vi "test-Vision-Utils-Test1.vi"() -> (3 "All Passed":bool)   [LabVIEW 2019]
uses:
  <vilib>/Rock Robotics/WPI/ThirdParty/JAS_Junk/TrajLib/Trajectory_Library.lvlib
panel:
  out "Dist To Targ 4":bool
  out "Dist To Targ 3":bool
  out "Dist To Targ 2":bool
  out "Dist To Targ 1":bool
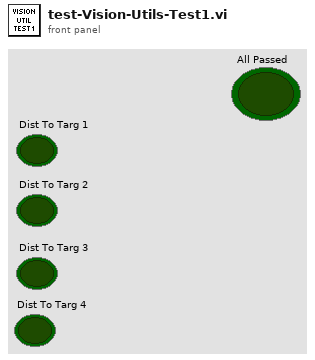
[diagram p1: front panel]
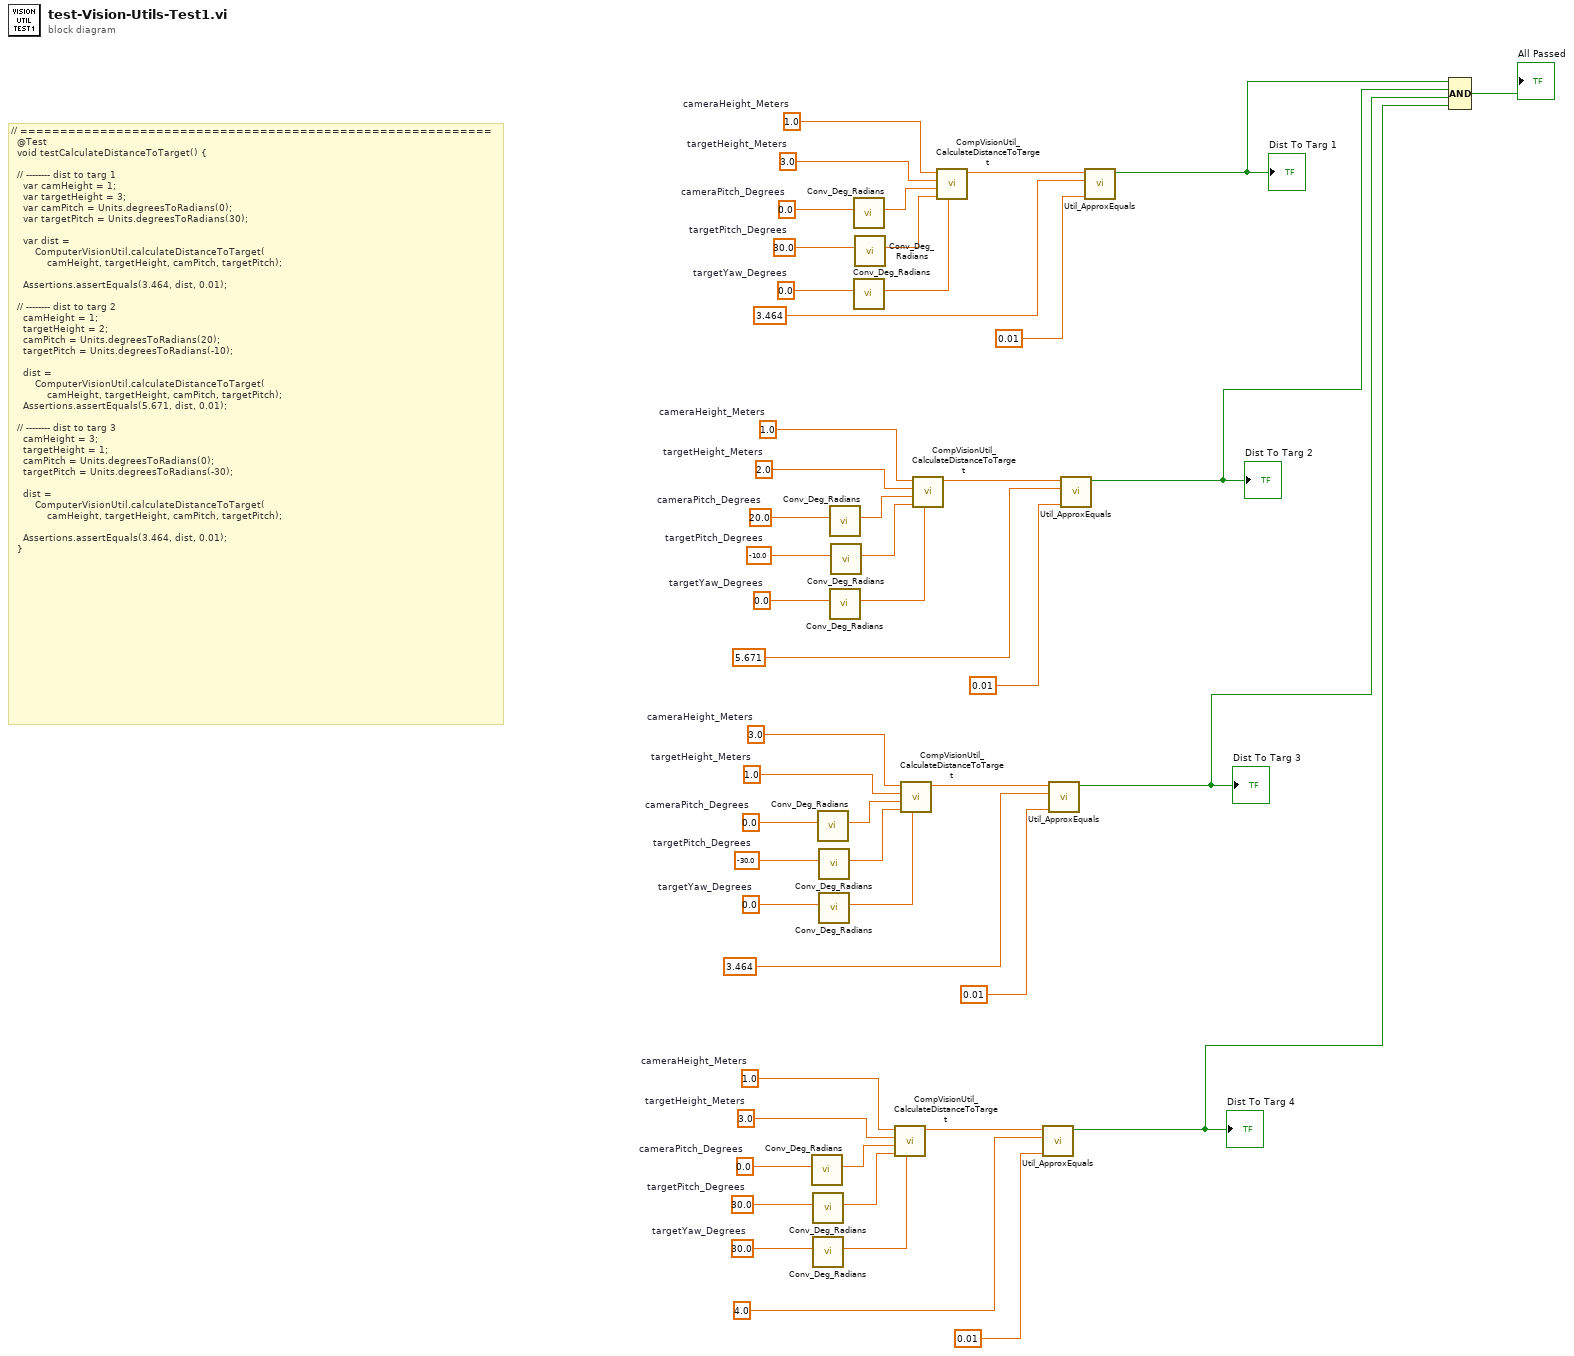
[diagram p0: block diagram]
diagram:
  w3 = 30.0  # targetYaw_Degrees
  w11 = 1.0  # cameraHeight_Meters
  w12 = 3.0  # targetHeight_Meters
  w10 = 0.0  # cameraPitch_Degrees
  w9 = 30.0  # targetPitch_Degrees
  w14 = 0.0  # targetYaw_Degrees
  w16 = 0.0  # targetYaw_Degrees
  w18 = 0.0  # targetYaw_Degrees
  w28 = 3.0  # cameraHeight_Meters
  w29 = 1.0  # targetHeight_Meters
  w27 = 0.0  # cameraPitch_Degrees
  w26 = -30.0  # targetPitch_Degrees
  w37 = 1.0  # cameraHeight_Meters
  w38 = 2.0  # targetHeight_Meters
  w36 = 20.0  # cameraPitch_Degrees
  w35 = -10.0  # targetPitch_Degrees
  w46 = 1.0  # cameraHeight_Meters
  w47 = 3.0  # targetHeight_Meters
  w45 = 0.0  # cameraPitch_Degrees
  w44 = 30.0  # targetPitch_Degrees
  # "// ===========================================================\n  @Test\n  void testCalculateDistanceToTarget() {\n\n  // -------- dist to targ 1\n    var camHeight = 1;\n    var targetHeight = 3;\n    var camPitch = Units.degreesToRadians(0);\n    var targetPitch = Units.degreesToRadians(30);\n\n    var dist =\n        ComputerVisionUtil.calculateDistanceToTarget(\n            camHeight, targetHeight, camPitch, targetPitch);\n\n    Assertions.assertEquals(3.464, dist, 0.01);\n\n  // -------- dist to targ 2\n    camHeight = 1;\n    targetHeight = 2;\n    camPitch = Units.degreesToRadians(20);\n    targetPitch = Units.degreesToRadians(-10);\n\n    dist =\n        ComputerVisionUtil.calculateDistanceToTarget(\n            camHeight, targetHeight, camPitch, targetPitch);\n    Assertions.assertEquals(5.671, dist, 0.01);\n\n  // -------- dist to targ 3\n    camHeight = 3;\n    targetHeight = 1;\n    camPitch = Units.degreesToRadians(0);\n    targetPitch = Units.degreesToRadians(-30);\n\n    dist =\n        ComputerVisionUtil.calculateDistanceToTarget(\n            camHeight, targetHeight, camPitch, targetPitch);\n\n    Assertions.assertEquals(3.464, dist, 0.01);\n  }"
  n1 = call <vilib>:"Conv_Deg_Radians.vi"("Degress"=w10) -> ("Radians"=w8:dbl)  [unwired: 10 in]
  n2 = call <vilib>:"Conv_Deg_Radians.vi"("Degress"=w9) -> ("Radians"=w7:dbl)  [unwired: 10 in]
  n3 = call <vilib>:"Conv_Deg_Radians.vi"("Degress"=w3) -> ("Radians"=w2:dbl)  [unwired: 10 in]
  n4 = call <vilib>:"Conv_Deg_Radians.vi"("Degress"=w27) -> ("Radians"=w25:dbl)  [unwired: 10 in]
  n5 = call <vilib>:"Conv_Deg_Radians.vi"("Degress"=w26) -> ("Radians"=w24:dbl)  [unwired: 10 in]
  n6 = call <vilib>:"Conv_Deg_Radians.vi"("Degress"=w14) -> ("Radians"=w13:dbl)  [unwired: 10 in]
  n7 = call <vilib>:"Conv_Deg_Radians.vi"("Degress"=w36) -> ("Radians"=w34:dbl)  [unwired: 10 in]
  n8 = call <vilib>:"Conv_Deg_Radians.vi"("Degress"=w16) -> ("Radians"=w15:dbl)  [unwired: 10 in]
  n9 = call <vilib>:"Conv_Deg_Radians.vi"("Degress"=w35) -> ("Radians"=w33:dbl)  [unwired: 10 in]
  n10 = call <vilib>:"Conv_Deg_Radians.vi"("Degress"=w45) -> ("Radians"=w43:dbl)  [unwired: 10 in]
  n11 = call <vilib>:"Conv_Deg_Radians.vi"("Degress"=w18) -> ("Radians"=w17:dbl)  [unwired: 10 in]
  n12 = call <vilib>:"Conv_Deg_Radians.vi"("Degress"=w44) -> ("Radians"=w42:dbl)  [unwired: 10 in]
  n13 = call <vilib>:"CompVisionUtil_CalculateDistanceToTarget.vi"("TargetYawRadians"=w2, "targetPitch_Radians"=w7, "cameraPitch_Radians"=w8, "targetHeight_Meters"=w12, "cameraHeight_Meters"=w11) -> ("DistanceToTarget_Meters"=w6:dbl)  [unwired: 6 in]
  n14 = call <vilib>:"CompVisionUtil_CalculateDistanceToTarget.vi"("TargetYawRadians"=w13, "targetPitch_Radians"=w24, "cameraPitch_Radians"=w25, "targetHeight_Meters"=w29, "cameraHeight_Meters"=w28) -> ("DistanceToTarget_Meters"=w23:dbl)  [unwired: 6 in]
  n15 = call <vilib>:"CompVisionUtil_CalculateDistanceToTarget.vi"("TargetYawRadians"=w15, "targetPitch_Radians"=w33, "cameraPitch_Radians"=w34, "targetHeight_Meters"=w38, "cameraHeight_Meters"=w37) -> ("DistanceToTarget_Meters"=w32:dbl)  [unwired: 6 in]
  n16 = call <vilib>:"CompVisionUtil_CalculateDistanceToTarget.vi"("TargetYawRadians"=w17, "targetPitch_Radians"=w42, "cameraPitch_Radians"=w43, "targetHeight_Meters"=w47, "cameraHeight_Meters"=w46) -> ("DistanceToTarget_Meters"=w41:dbl)  [unwired: 6 in]
  n17 = call <vilib>:"Util_ApproxEquals.vi"("Tolerance"=0.01, "Value 2"=4.0, "Value 1"=w6) -> ("ApproxEquals"=w1:bool)  [unwired: 8 in]
  "Dist To Targ 4" <- w1
  n18 = call <vilib>:"Util_ApproxEquals.vi"("Tolerance"=0.01, "Value 2"=3.464, "Value 1"=w23) -> ("ApproxEquals"=w19:bool)  [unwired: 8 in]
  "Dist To Targ 3" <- w19
  n19 = call <vilib>:"Util_ApproxEquals.vi"("Tolerance"=0.01, "Value 2"=5.671, "Value 1"=w32) -> ("ApproxEquals"=w20:bool)  [unwired: 8 in]
  "Dist To Targ 2" <- w20
  n20 = call <vilib>:"Util_ApproxEquals.vi"("Tolerance"=0.01, "Value 2"=3.464, "Value 1"=w41) -> ("ApproxEquals"=w49:bool)  [unwired: 8 in]
  "Dist To Targ 1" <- w49
  n21 = Compound Arithmetic op=AND(w49, w20, w19, w1) -> (→"All Passed":bool)
